vi "FlussdichteAnpassen.vi"(8 "Error in":errorcluster, 9 "Globale Variablen":T1, 10 "GUI Data":T3, 11 "GUI Einstellungen":T2) -> (0 "Error out":errorcluster, 1 "Globale Variablen out":T1, 2 "GUI Data out":T3, 3 "GUI Einstellungen out":T2)   [LabVIEW 2016]
doc: "Übergibt dem VI Anpassung die Spannungswerte. Die Spannungswerte werden in 2V, 1V, 0,5V, 0,1V, 0,05V, 0,02V Schritten an das VI übergeben. Es uebernimmt somit die Schrittweitenvorgabe fuer den Regelungsalgorithmus in Anpassung.vi\n\nBricht den Vorgang ab sobald die gewünschte Spannung bzw. Flussdichte erreicht wird, oder die Grenzen des Frequenzgenerators erreicht sind."
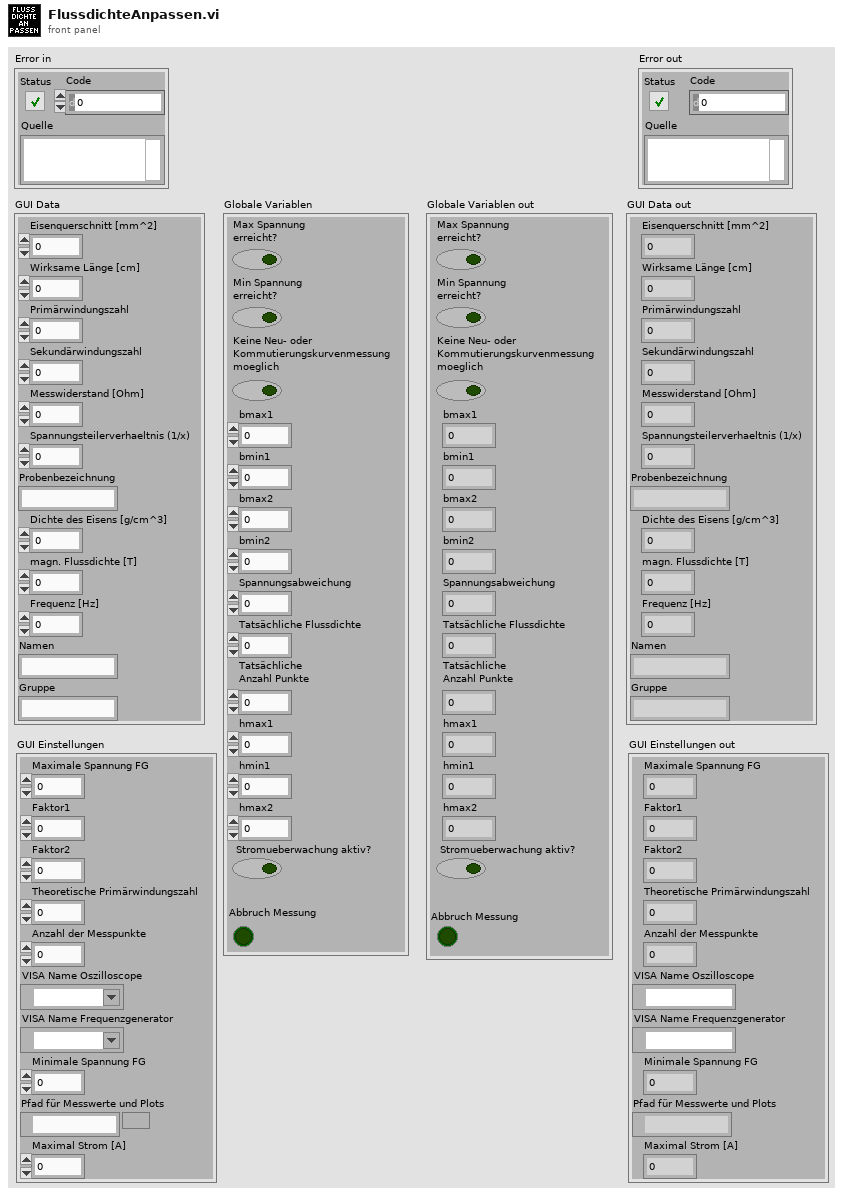
[diagram p1: front panel]
types:
  T1 = cluster{"Max Spannung\nerreicht?":bool, "Min Spannung\nerreicht?":bool, "Keine Neu- oder\nKommutierungskurvenmessung\nmoeglich":bool, "bmax1":dbl, "bmin1":dbl, "bmax2":dbl, "bmin2":dbl, "Spannungsabweichung":dbl, "Tatsächliche Flussdichte":dbl, "Tatsächliche \nAnzahl Punkte":dbl, "hmax1":dbl, "hmin1":dbl, "hmax2":dbl, " Stromueberwachung aktiv?":bool, "Abbruch Messung":bool}
  T2 = cluster{"Maximale Spannung FG":dbl, "Faktor1":dbl, "Faktor2":dbl, "Theoretische Primärwindungszahl":dbl, "Anzahl der Messpunkte":i32, "VISA Name Oszilloscope":refnum<visa-resource-name>, "VISA Name Frequenzgenerator":refnum<visa-resource-name>, "Minimale Spannung FG":dbl, "Pfad für Messwerte und Plots":path, "Maximal Strom [A] ":dbl}
  T3 = cluster{"Eisenquerschnitt [mm^2]":dbl, "Wirksame Länge [cm]":dbl, "Primärwindungszahl":dbl, "Sekundärwindungszahl":dbl, "Messwiderstand [Ohm]":dbl, "Spannungsteilerverhaeltnis (1/x)":dbl, "Probenbezeichnung":string, "Dichte des Eisens [g/cm^3]":dbl, "magn. Flussdichte [T]":dbl, "Frequenz [Hz]":dbl, "Namen":string, "Gruppe":string}
  T4 = enum16{"Add_2V", "Add_1V", "Add_0.5V", "Add_0.1V", "Add_0.05V", "Add_0.02V", ""}
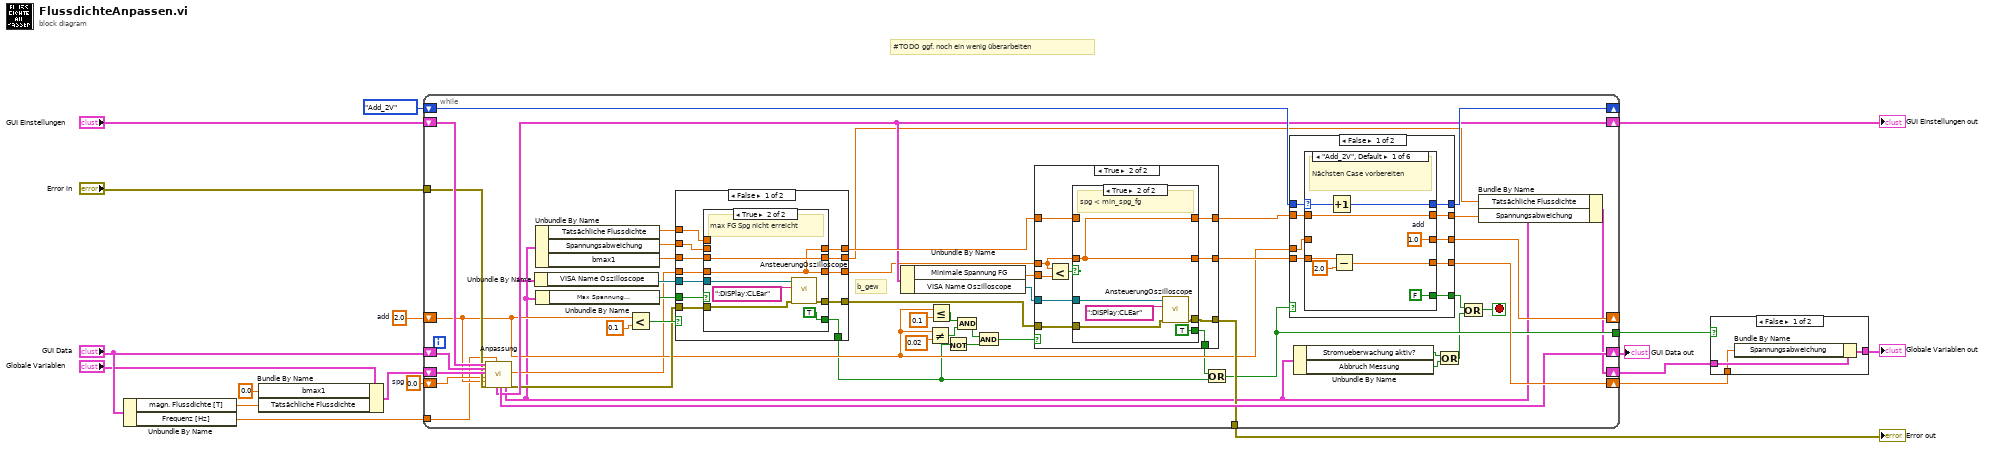
[diagram p0: block diagram]
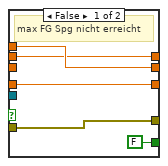
[diagram p2: hidden frame]
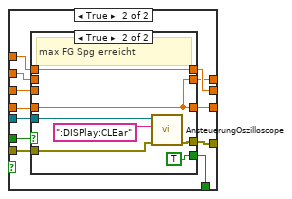
[diagram p3: hidden frame]
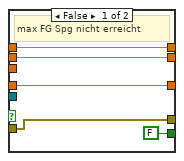
[diagram p4: hidden frame]
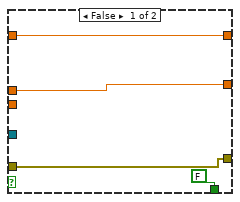
[diagram p5: hidden frame]
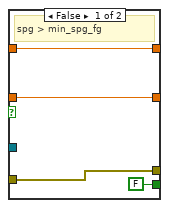
[diagram p6: hidden frame]
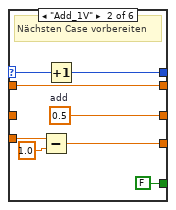
[diagram p7: hidden frame]
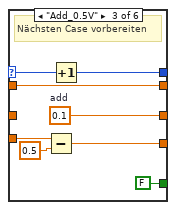
[diagram p8: hidden frame]
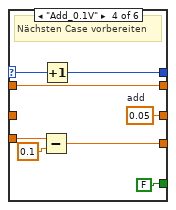
[diagram p9: hidden frame]
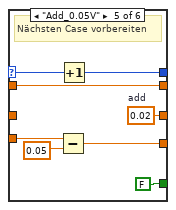
[diagram p10: hidden frame]
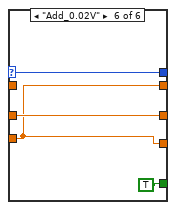
[diagram p11: hidden frame]
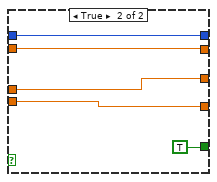
[diagram p12: hidden frame]
diagram:
  w16 = 0.0  # spg
  w17 = 2.0  # add
  # "#TODO ggf. noch ein wenig überarbeiten"
  n1 = Unbundle By Name("GUI Data") -> ("magn. Flussdichte [T]"=w11:dbl, "Frequenz [Hz]"=w7:dbl)
  n2 = Bundle By Name(cluster="Globale Variablen", "bmax1"=0.0, "Tatsächliche Flussdichte"=w11) -> (w13:T1)
  n3 = while {
    shift-right: [w66] -> _
    shift-left: T4."Add_2V" -> [w67]
    shift-right: [w65] -> _
    shift-left: w17 -> [w39]
    shift-right: [w64] -> w8
    shift-left: w16 -> [w58]
    tunnel: "Error in" -> [w60]
    shift-right: [w48] -> w5
    shift-left: "GUI Einstellungen" -> [w63]
    shift-right: [w59] -> w14
    shift-left: "GUI Data" -> [w62]
    shift-right: [w25] -> w1
    shift-left: w13 -> [w61]
    tunnel: [w45] -> w10
    tunnel: [w35] -> w9
    tunnel: w7 -> [w27]
    stop <- w22 stop-if-true
    # "b_gew"
    n4 = call "Anpassung.vi"("GUI Einstellungen"=w63, "GUI Data"=w62, "Globale Variablen"=w61, "Spannung (0)"=w58, "Add (0)"=w39, "Error in"=w60, "Frequency (1000 Hz)"=w27) -> ("GUI Einstellungen out"=w48:T2, "GUI data out"=w59:T3, "Globale Variablen out"=w24:T1, "Spannung"=w34:dbl, "Error out"=w46:errorcluster)  [unwired: 8 in]
    n5 = Unbundle By Name(w48) -> ("VISA Name Oszilloscope"=w47:refnum<visa-resource-name>)
    n6 = Unbundle By Name(w24) -> ("Tatsächliche Flussdichte"=w57:dbl, "Spannungsabweichung"=w32:dbl, "bmax1"=w31:dbl)
    n7 = Unbundle By Name(w24) -> ("Max Spannung\nerreicht?"=w56:bool)
    n8 = Less?(x=w39, y=0.1) -> (x < y?=w54:bool)
    n9 = case shown="False" w54 {
      tunnel: w56 -> [w68 w92]
      tunnel: w31 -> [w76 w103]
      tunnel: [w75 w102] -> w28
      tunnel: w34 -> [w79 w101]
      tunnel: [w78 w100] -> w51
      tunnel: w57 -> [w71 w99]
      tunnel: w32 -> [w77 w93]
      tunnel: [w74 w98] -> w49
      tunnel: w47 -> [w72 w97]
      tunnel: w46 -> [w73 w96]
      tunnel: [w70 w95] -> w36
      tunnel: [w69 w94] -> w33
      frame False {
        n10 = case shown="True" w68 {
          tunnel: w79 -> [w81 w85]
          tunnel: [w80 w85] -> w78
          tunnel: w77 -> [w80 _]
          tunnel: w76 -> [_ w91]
          tunnel: [w84 w91] -> w75
          tunnel: [w82 w89] -> w74
          tunnel: w73 -> [w82 w88]
          tunnel: w72 -> [_ w87]
          tunnel: w71 -> [w84 _]
          tunnel: [FALSE TRUE] -> w70
          tunnel: [w81 w85] -> w69
          frame False {
            # "max FG Spg nicht erreicht"
          }
          frame True {
            # "max FG Spg nicht erreicht"
            n11 = call "AnsteuerungOszilloscope.vi"("Error_in"=w88, "Eingangs-String"=":DISPlay:CLEar", "VISA Name OZ in(OZ)"=w87) -> ("Error_out"=w89:errorcluster)  [unwired: 6 in, 2 out]
          }
        }
      }
      frame True {
        n12 = case shown="True" w92 {
          tunnel: w103 -> [_ _]
          tunnel: [w108 w111] -> w102
          tunnel: w101 -> [w105 w109]
          tunnel: [w104 w109] -> w100
          tunnel: w99 -> [w108 w111]
          tunnel: w93 -> [w104 _]
          tunnel: [w107 w114] -> w98
          tunnel: w97 -> [_ w113]
          tunnel: w96 -> [w107 w112]
          tunnel: [FALSE TRUE] -> w95
          tunnel: [w105 w109] -> w94
          frame False {
            # "max FG Spg nicht erreicht"
          }
          frame True {
            # "max FG Spg erreicht"
            n13 = call "AnsteuerungOszilloscope.vi"("Error_in"=w112, "Eingangs-String"=":DISPlay:CLEar", "VISA Name OZ in(OZ)"=w113) -> ("Error_out"=w114:errorcluster)  [unwired: 6 in, 2 out]
          }
        }
      }
    }
    n14 = Unbundle By Name(w48) -> ("Minimale Spannung FG"=w52:dbl, "VISA Name Oszilloscope"=w50:refnum<visa-resource-name>)
    n15 = Not Equal?(x=w39, y=0.02) -> (x != y?=w41:bool)
    n16 = Less Or Equal?(x=w39, y=0.1) -> (x <= y?=w42:bool)
    n17 = Not(x=w36) -> (.not. x?=w30:bool)
    n18 = And(x=w42, y=w41) -> (x .and. y?=w29:bool)
    n19 = And(x=w29, y=w30) -> (x .and. y?=w38:bool)
    n20 = case shown="True" w38 {
      tunnel: w33 -> [w119 w125]
      tunnel: w52 -> [_ w129]
      tunnel: w51 -> [w118 w126]
      tunnel: [w118 w127] -> w44
      tunnel: w50 -> [_ w124]
      tunnel: w49 -> [w116 w123]
      tunnel: [w116 w122] -> w45
      tunnel: [w119 w121] -> w43
      tunnel: [FALSE w120] -> w37
      frame False {
      }
      frame True {
        n21 = Less?(x=w125, y=w129) -> (x < y?=w128:bool)
        n22 = case shown="True" w128 {
          tunnel: [w133 w135] -> w127
          tunnel: w126 -> [w133 _]
          tunnel: w125 -> [w131 w135]
          tunnel: w124 -> [_ w139]
          tunnel: w123 -> [w132 w137]
          tunnel: [w132 w136] -> w122
          tunnel: [w131 w135] -> w121
          tunnel: [FALSE TRUE] -> w120
          frame False {
            # "spg > min_spg_fg"
          }
          frame True {
            # "spg < min_spg_fg"
            n23 = call "AnsteuerungOszilloscope.vi"("Error_in"=w137, "Eingangs-String"=":DISPlay:CLEar", "VISA Name OZ in(OZ)"=w139) -> ("Error_out"=w136:errorcluster)  [unwired: 6 in, 2 out]
          }
        }
      }
    }
    n24 = Or(x=w37, y=w36) -> (x .or. y?=w35:bool)
    n25 = case shown="False" w35 {
      tunnel: w67 -> [w142 w194]
      tunnel: [w148 w194] -> w66
      tunnel: [w147 w195] -> w65
      tunnel: [w146 w196] -> w64
      tunnel: w44 -> [w145 w197]
      tunnel: [w144 w197] -> w26
      tunnel: w43 -> [w143 w196]
      tunnel: [w141 TRUE] -> w23
      tunnel: w39 -> [w140 w195]
      frame False {
        n26 = case shown="\"Add_2V\", Default" w142 {
          selector: w142 -> [w156 w164 w172 w180 w188 w192]
          tunnel: [w155 w163 w171 w179 w187 w192] -> w148
          tunnel: [w154 w159 w167 w175 w183 w190] -> w147
          tunnel: [w152 w160 w168 w176 w184 w189] -> w146
          tunnel: w143 -> [w151 w161 w169 w177 w185 w189]
          tunnel: [FALSE FALSE FALSE FALSE FALSE TRUE] -> w141
          tunnel: w140 -> [_ _ _ _ _ w190]
          tunnel: w145 -> [w150 w158 w166 w174 w182 _]
          tunnel: [w150 w158 w166 w174 w182 w189] -> w144
          frame "Add_2V", Default {
            w154 = 1.0  # add
            # "Nächsten Case vorbereiten"
            n27 = Increment(x=w156) -> (x+1=w155:T4)
            n28 = Subtract(x=w151, y=2.0 ("spg")) -> (x-y=w152:dbl)
          }
          frame "Add_1V" {
            w159 = 0.5  # add
            # "Nächsten Case vorbereiten"
            n29 = Subtract(x=w161, y=1.0 ("spg")) -> (x-y=w160:dbl)
            n30 = Increment(x=w164) -> (x+1=w163:T4)
          }
          frame "Add_0.5V" {
            w167 = 0.1  # add
            # "Nächsten Case vorbereiten"
            n31 = Subtract(x=w169, y=0.5 ("spg")) -> (x-y=w168:dbl)
            n32 = Increment(x=w172) -> (x+1=w171:T4)
          }
          frame "Add_0.1V" {
            w175 = 0.05  # add
            # "Nächsten Case vorbereiten"
            n33 = Subtract(x=w177, y=0.1 ("spg")) -> (x-y=w176:dbl)
            n34 = Increment(x=w180) -> (x+1=w179:T4)
          }
          frame "Add_0.05V" {
            w183 = 0.02  # add
            # "Nächsten Case vorbereiten"
            n35 = Subtract(x=w185, y=0.05 ("spg")) -> (x-y=w184:dbl)
            n36 = Increment(x=w188) -> (x+1=w187:T4)
          }
          frame "Add_0.02V" {
          }
        }
      }
      frame True {
      }
    }
    n37 = Unbundle By Name(w24) -> ("Stromueberwachung aktiv?"=w20:bool, "Abbruch Messung"=w19:bool)
    n38 = Or(x=w20, y=w19) -> (x .or. y?=w21:bool)
    n39 = Or(x=w23, y=w21) -> (x .or. y?=w22:bool)
    n40 = Bundle By Name(cluster=w24, "Tatsächliche Flussdichte"=w28, "Spannungsabweichung"=w26) -> (w25:T1)
  }
  "GUI Data out" <- w14
  "Error out" <- w10
  "GUI Einstellungen out" <- w5
  n41 = case shown="False" w9 {
    tunnel: [w200 w201] -> w3
    tunnel: w8 -> [w198 _]
    tunnel: w1 -> [w199 w201]
    frame False {
      n42 = Bundle By Name(cluster=w199, "Spannungsabweichung"=w198) -> (w200:T1)
    }
    frame True {
    }
  }
  "Globale Variablen out" <- w3
